vi "Ultimate randomizator 3000.vi"(10 "Signal":dbl) -> (2 "Sign+Noise":dbl)   [LabVIEW 2020]
panel:
  # "[Prototype]"
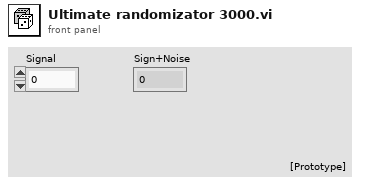
[diagram p1: front panel]
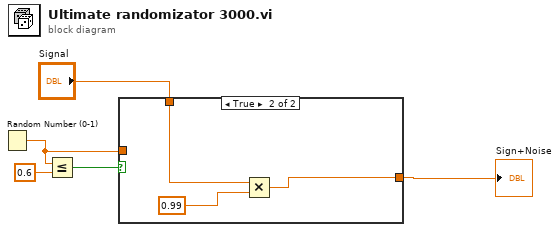
[diagram p0: block diagram]
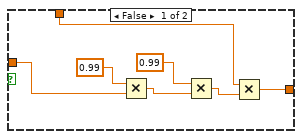
[diagram p2: hidden frame]
diagram:
  n1 = Random Number (0-1)() -> (number: 0 to 1=w5:dbl)
  n2 = Less Or Equal?(x=w5, y=0.6) -> (x <= y?=w2:bool)
  n3 = case shown="True" w2 {
    tunnel: "Signal" -> [w6 w15]
    tunnel: [w8 w13] -> w4
    tunnel: w5 -> [w12 _]
    frame False {
      n4 = Multiply(x=0.99, y=w12) -> (x*y=w10:dbl)
      n5 = Multiply(x=0.99, y=w10) -> (x*y=w7:dbl)
      n6 = Multiply(x=w6, y=w7) -> (x*y=w8:dbl)
    }
    frame True {
      n7 = Multiply(x=w15, y=0.99) -> (x*y=w13:dbl)
    }
  }
  "Sign+Noise" <- w4
